vi "Async Start video from CamServer (for web monitoring).vi"(1 "Quality":i32=750 min=0 max=1000, 2 "Camera":T1="Travcam") -> (0 "Error out":errorcluster)   [LabVIEW 2015]
uses:
  Camera enum/Camera enum.ctl
panel:
  # "PN 21/08/15"
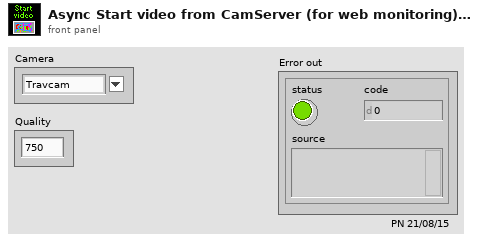
[diagram p1: front panel]
types:
  T1 = typedef "Camera enum.ctl" = string
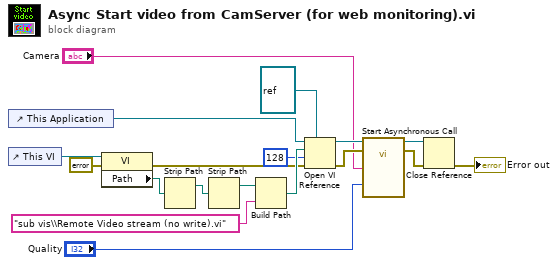
[diagram p0: block diagram]
diagram:
  n1 = control-ref of="This Application"() -> (w13:refnum<vi>)
  n2 = control-ref of="This VI"() -> (w18:refnum<vi>)
  n3 = property class="VI"(reference=w18, error in=errorcluster {"status"=FALSE, "code"=0, "source"=""} ("error in (no error)")) -> (error out=w15:errorcluster, "Path"=w11:path)  [unwired: 1 out]
  n4 = Strip Path(path=w11) -> (stripped path=w3:path)  [unwired: 1 out]
  n5 = Strip Path(path=w3) -> (stripped path=w2:path)  [unwired: 1 out]
  n6 = Build Path(base path=w2, name or relative path="sub vis\\Remote Video stream (no write).vi") -> (appended path=w16:path)
  n7 = Open VI Reference(type specifier VI Refnum (for type only)=refnum<vi> refnum, application reference (local)=w13, vi path=w16, options=128, error in (no error)=w15) -> (vi reference=w10:refnum<vi>, error out=w9:errorcluster)  [unwired: 1 in]
  n8 = call-by-ref "Start Asynchronous Call"(reference=w10, error in=w9, "Quality"="Quality", "Camera"="Camera") -> (reference out=w6:refnum<vi>, error out=w5:errorcluster)  [unwired: 1 out]
  n9 = Close Reference(reference=w6, error in (no error)=w5) -> (error out=→"Error out":errorcluster)
